vi "CCD Handle.vi"(11 "簇":T2) -> ()   [LabVIEW 2018]
uses:
  <vilib>/userdefined/High Color/IMAQdx.ctl
  <vilib>/vision/Image Controls.llb/IMAQ Image.ctl
  <vilib>/vision/driver/NI_Vision_Acquisition_Software.lvlib
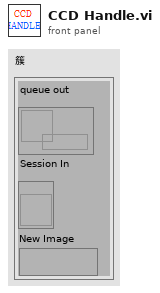
[diagram p1: front panel]
types:
  T1 = typedef "IMAQ Image.ctl" = refnum<image>
  T2 = cluster{"queue out":refnum<queue>, "Session In":refnum<vi>, "New Image":T1}
  T3 = typedef "IMAQdx.ctl" = refnum<k21>
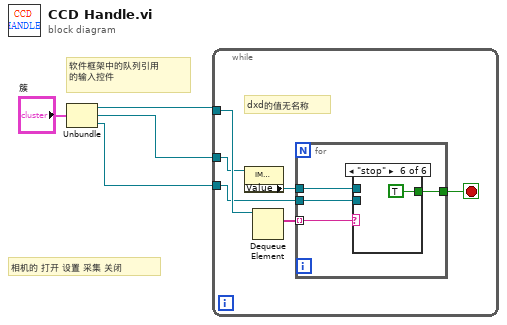
[diagram p0: block diagram]
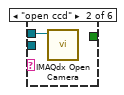
[diagram p3: hidden frame]
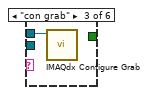
[diagram p4: hidden frame]
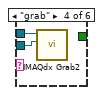
[diagram p5: hidden frame]
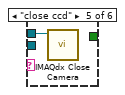
[diagram p6: hidden frame]
diagram:
  # "相机的 打开 设置 采集 关闭"
  # "软件框架中的队列引用\n的输入控件"
  n1 = Unbundle("簇") -> ("queue out"=w3:refnum<queue>, "Session In"=w2:refnum<vi>, "New Image"=w1:T1)
  n2 = while {
    tunnel: w3 -> [w10]
    tunnel: w2 -> [w6]
    tunnel: w1 -> [w8]
    stop <- w7 stop-if-true
    # "dxd的值无名称"
    n3 = property class="IMAQdx (严格)"(reference=w6) -> ("Value"=w5:T3)  [unwired: 1 in, 2 out]
    n4 = Dequeue Element(queue=w10) -> (element=w9:string[])  [unwired: 2 in, 3 out]
    n5 = for {
      tunnel: w9 -> [w14] mode=indexing
      tunnel: w5 -> [w13]
      tunnel: w8 -> [w12]
      tunnel: [w11] -> w7
      n6 = case shown="\"stop\"" w14 {
        tunnel: w13 -> [_ w15 w16 w18 w19 _]
        tunnel: w12 -> [_ _ _ w17 _ _]
        tunnel: [_ _ _ _ _ TRUE] -> w11
        frame "假", Default {
        }
        frame "open ccd" {
          n7 = call <vilib>:"IMAQdx Open Camera.vi"("Session In"=w15) -> ()  [unwired: 9 in, 2 out]
        }
        frame "con grab" {
          n8 = call <vilib>:"IMAQdx Configure Grab.vi"("Session In"=w16) -> ()  [unwired: 9 in, 2 out]
        }
        frame "grab" {
          n9 = call <vilib>:"IMAQdx Grab2.vi"("Image In"=w17, "Session In"=w18) -> ()  [unwired: 6 in, 4 out]
        }
        frame "close ccd" {
          n10 = call <vilib>:"IMAQdx Close Camera.vi"("Session In"=w19) -> ()  [unwired: 10 in, 1 out]
        }
        frame "stop" {
        }
      }
    }
  }
